vi "countrate_viewer_mpix.vi"() -> ()   [LabVIEW 2022 SP3]
uses:
  af06e324-2b0b-4744-b8ce-6f47c907ae65.vi
  <vilib>/Comparison/Less/Less Functor/Less Functor.lvclass
panel:
  in  "Thscan Folder Path":path=path "C:/Users/User/OneDrive/measurements/mpix/2023-04-14_pommiary_RK_testowe_przed_RG/0050mA/7a_ikrum=  2; igm= 32; vt0=  s; vt1=   ; DIS_DYN_SW= ; MPR_en= ; bgshc_W= ; bgshc_N= ; bgshc_NW= ;"
  in  "Current":u16(ring)=1 items=["0050mA", "0100mA", "0150mA"]
  in  "Tab Control":enum32{"Single pixel", "Pixels ROI"}(tab)
  out "Counns_vs_Current":cluster{i32[], i32[]}(graph)
  out "SP_Thscans":i32[][](graph)
  out "ROI_Thscans":i32[][](graph)
  out "ROI Counns_vs_Current":cluster{"x":i32[], "y":i32[]}[](graph)
  out "Image":i32[][](graph)
  in  "ThScan_Load":bool
  in  "Exit":bool
  # "counts vs. current for single pixel for single vt"
  # "thscans of all currents for single pixel"
  # "counts vs. current for ROI pixels for single vt"
  # "thscans of ROI pixels for single current"
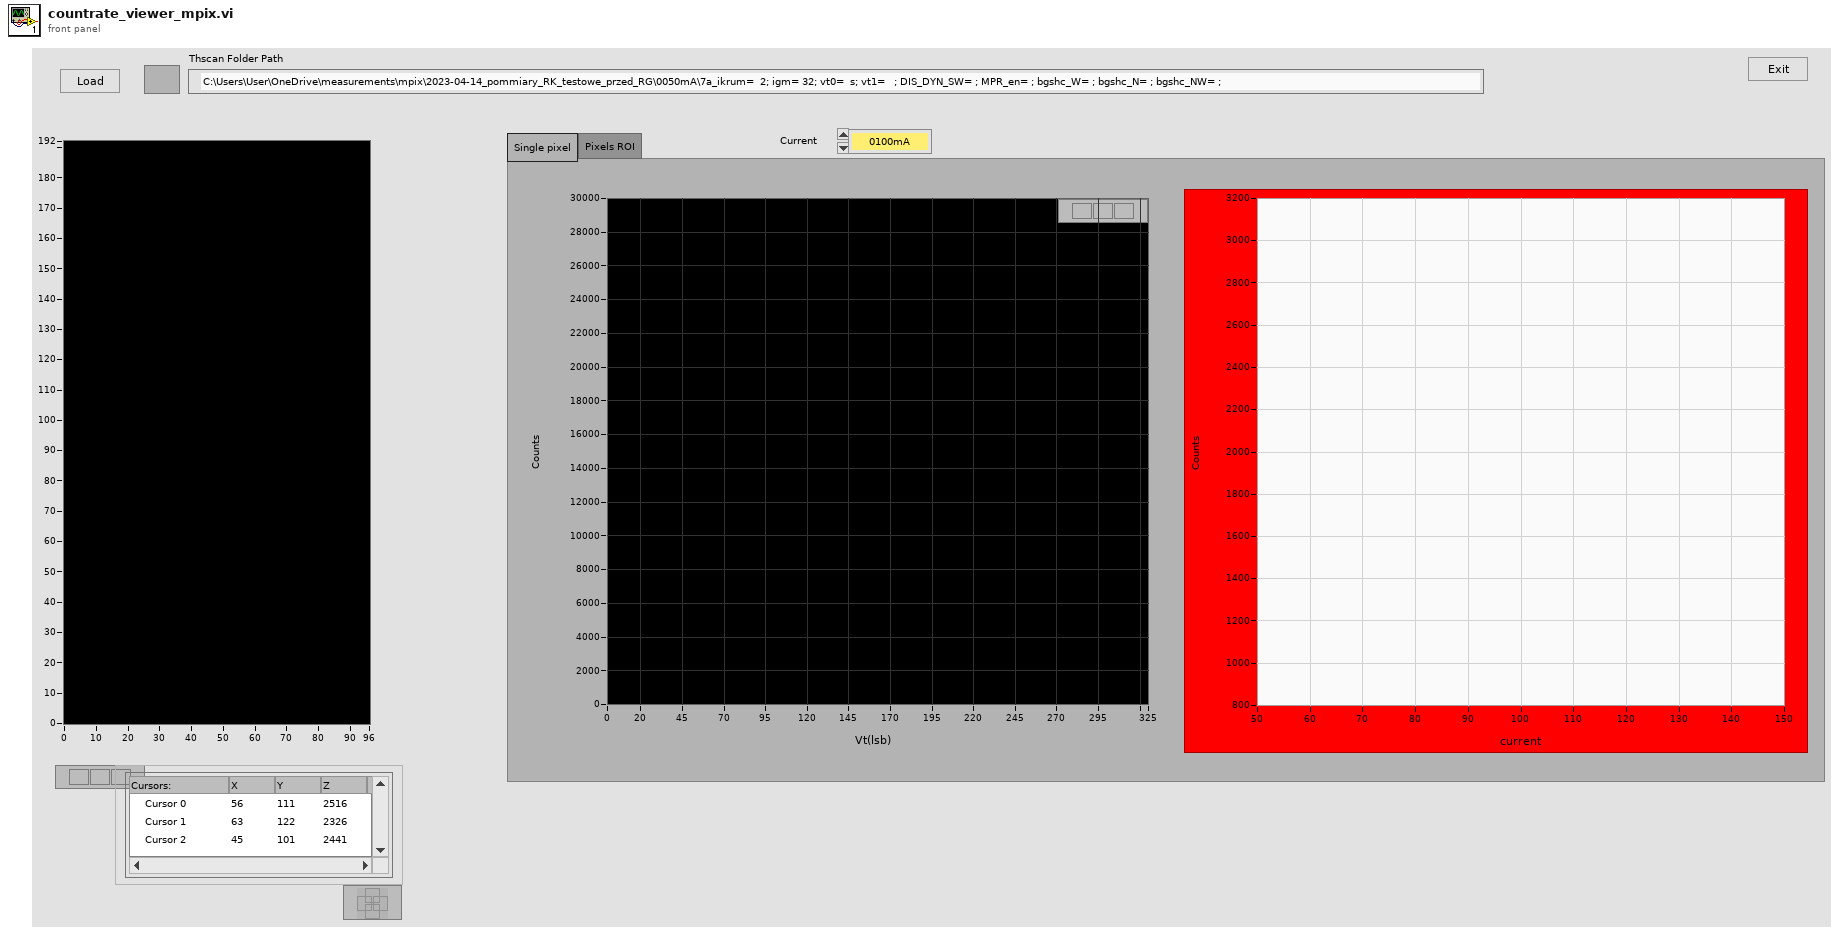
[diagram p1: front panel]
types:
  T1 = enum16{"big-endian, network order", "native, host order", "little-endian"}
  T2 = typedef "LVPointDoubleTypeDef.ctl" = cluster{"Cursor X":dbl, "Cursor Y":dbl}
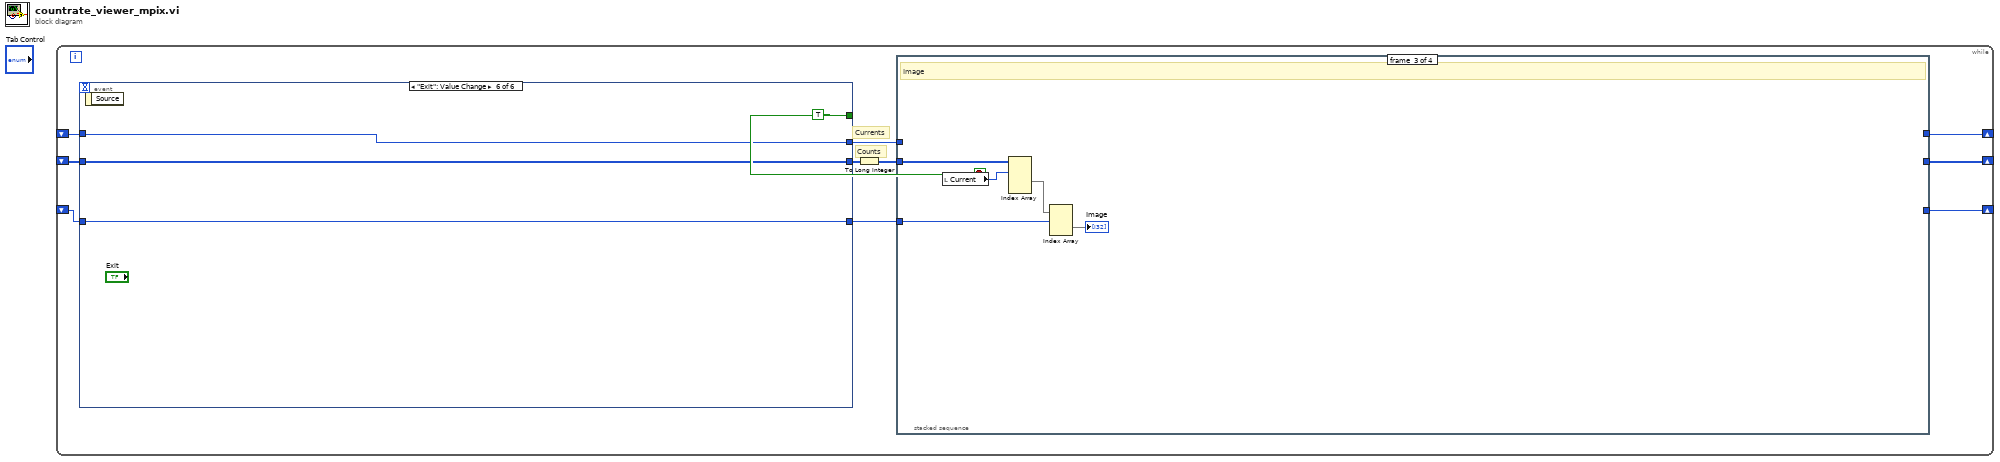
[diagram p0: block diagram]
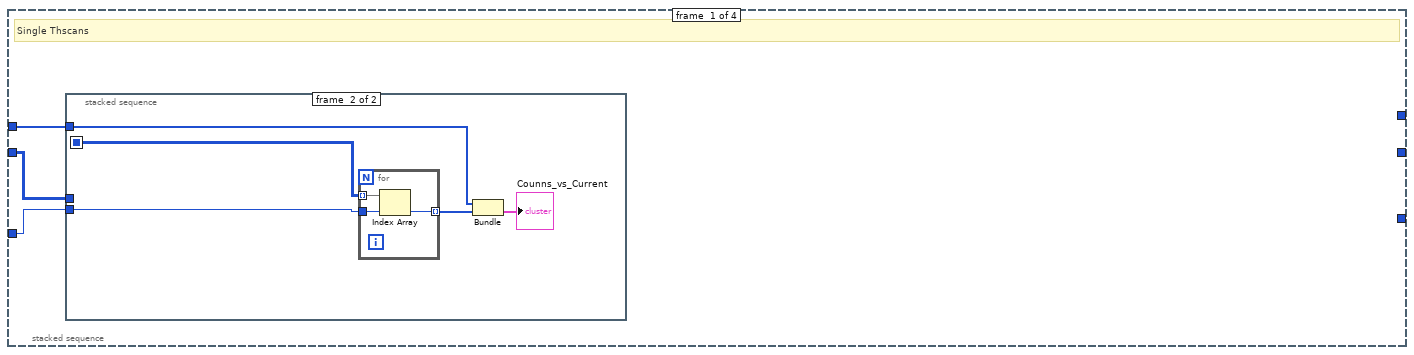
[diagram p2: hidden frame]
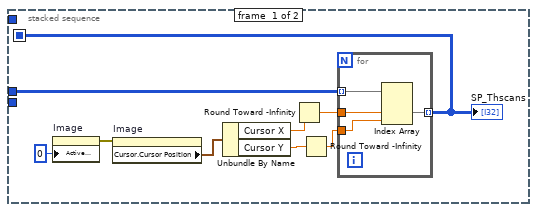
[diagram p3: hidden frame]
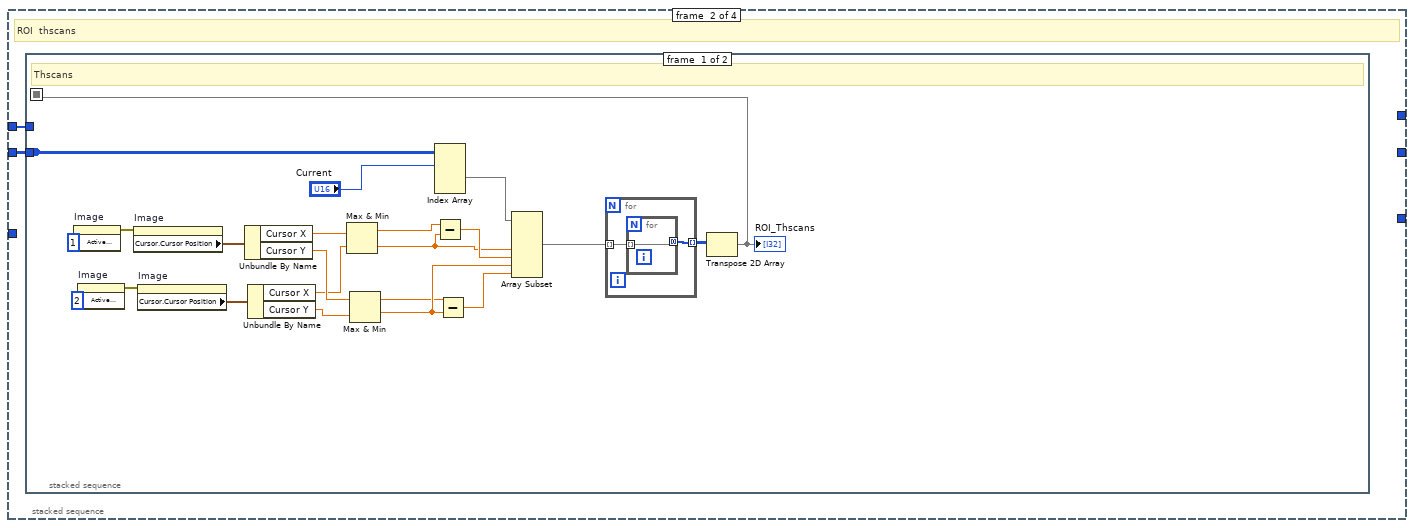
[diagram p4: hidden frame]
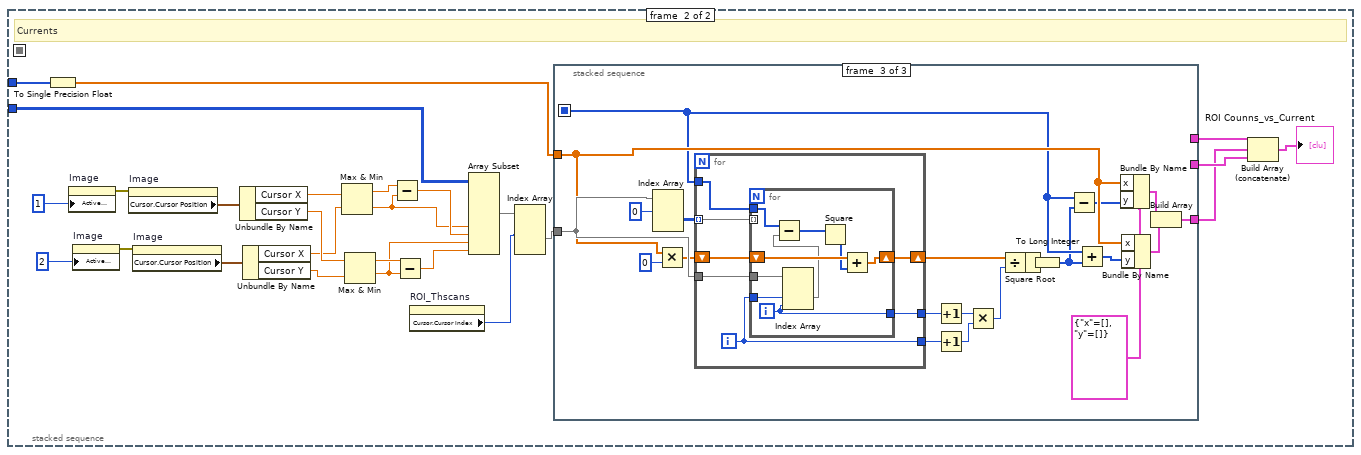
[diagram p5: hidden frame]
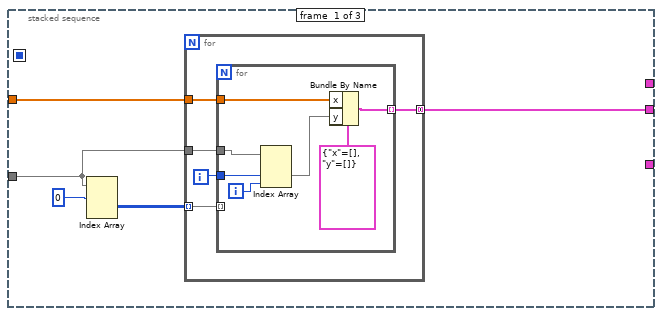
[diagram p6: hidden frame]
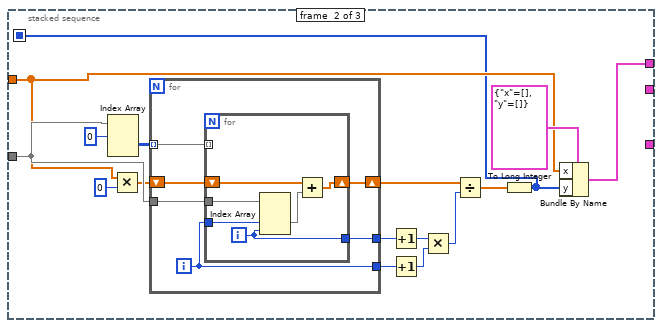
[diagram p7: hidden frame]
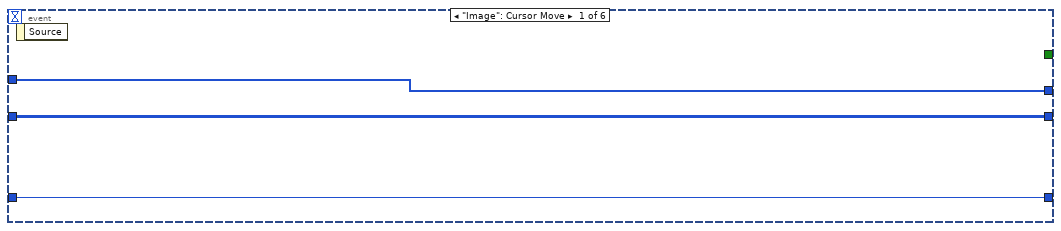
[diagram p9: hidden frame]
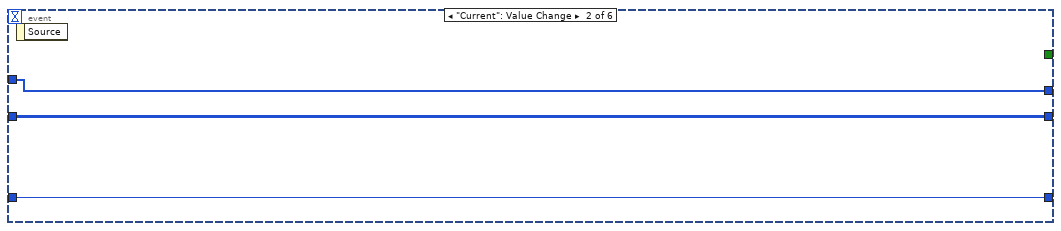
[diagram p10: hidden frame]
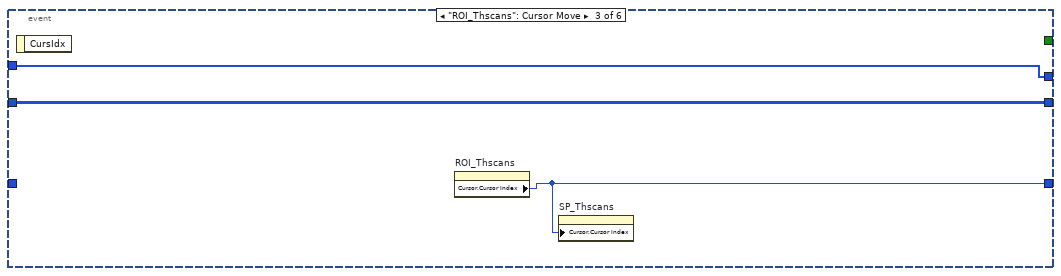
[diagram p11: hidden frame]
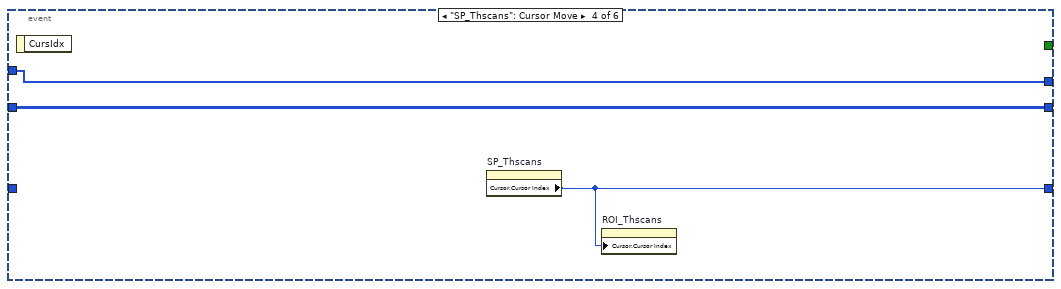
[diagram p12: hidden frame]
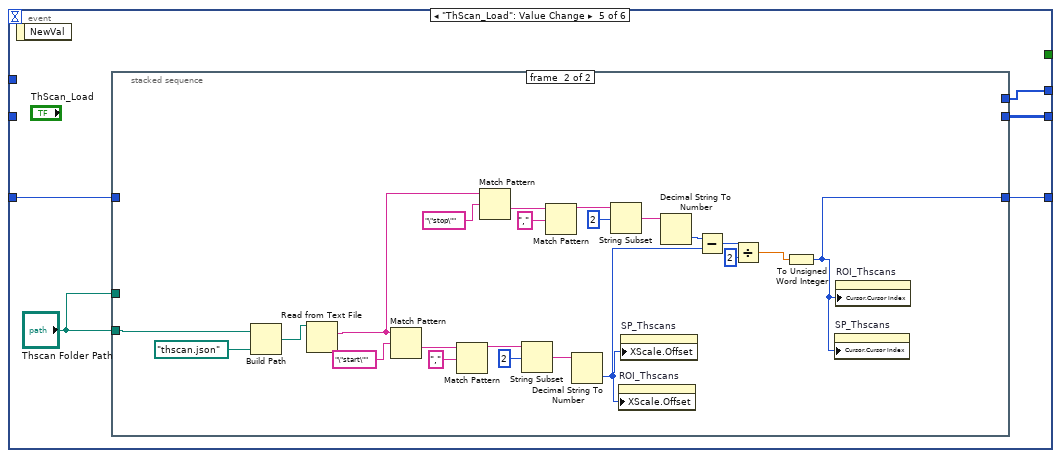
[diagram p13: hidden frame]
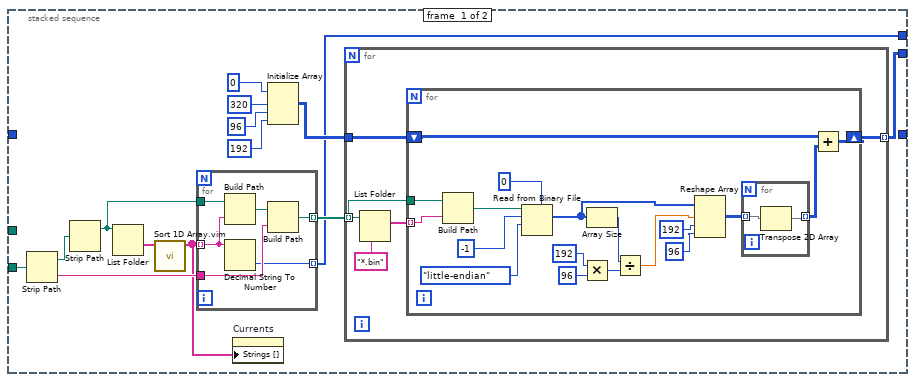
[diagram p14: hidden frame]
diagram:
  n1 = while {
    shift-right: [w8] -> _
    shift-left: _ -> [w10]
    shift-right: [w5] -> _
    shift-left: _ -> [w7]
    shift-right: [w2] -> _
    shift-left: _ -> [w1]
    stop <- w11 stop-if-true
    # "Counts"
    # "Currents"
    n2 = event shown="[5] \"Exit\": Value Change" {
      selector: _ -> [_ _ _ _ _ _]
      dyn-events: _ -> [_ _ _ _ _ _]
      timeout: _ -> [_ _ _ _ _ _]
      tunnel: [_ _ _ _ _ TRUE] -> w11
      tunnel: w10 -> [w182 w184 w188 w190 _ w266]
      tunnel: [w182 w184 w188 w190 w195 w266] -> w9
      tunnel: w7 -> [w181 w185 w187 w191 _ w265]
      tunnel: [w181 w185 w187 w191 w196 w265] -> w6
      tunnel: [w180 w183 w186 w189 w193 w264] -> w3
      tunnel: w1 -> [w180 w183 _ _ w192 w264]
      event "Image": Cursor Move {
        n3 = event-data() -> ()  [unwired: 1 in, 1 out]
      }
      event "Current": Value Change {
        n4 = event-data() -> ()  [unwired: 1 in, 1 out]
      }
      event "ROI_Thscans": Cursor Move {
        n5 = event-data() -> ()  [unwired: 1 in, 1 out]
        n6 = property on="ROI_Thscans" class="WFGraph (strict)"() -> ("Cursor.Cursor Index"=w186:i32)  [unwired: 2 in, 2 out]
        n7 = property on="SP_Thscans" class="WFGraph (strict)"("Cursor.Cursor Index"=w186) -> ()  [unwired: 2 in, 2 out]
      }
      event "SP_Thscans": Cursor Move {
        n8 = event-data() -> ()  [unwired: 1 in, 1 out]
        n9 = property on="SP_Thscans" class="WFGraph (strict)"() -> ("Cursor.Cursor Index"=w189:i32)  [unwired: 2 in, 2 out]
        n10 = property on="ROI_Thscans" class="WFGraph (strict)"("Cursor.Cursor Index"=w189) -> ()  [unwired: 2 in, 2 out]
      }
      event "ThScan_Load": Value Change {
        n11 = event-data() -> ()  [unwired: 1 in, 1 out]
        n12 = stacked-sequence {
          tunnel: [w200 _] -> w196
          tunnel: [w199 _] -> w195
          tunnel: "Thscan Folder Path" -> [w197 w255]
          tunnel: "Thscan Folder Path" -> [_ _]
          tunnel: [_ w243] -> w193
          tunnel: w192 -> [_ _]
          frame #0 {
            n13 = Strip Path(path=w197) -> (stripped path=w210:path, name=w208:string)
            n14 = Strip Path(path=w210) -> (stripped path=w207:path)  [unwired: 1 out]
            n15 = List Folder(path=w207) -> (folder names=w209:string[])  [unwired: 3 in, 3 out]
            n16 = call "Sort 1D Array.vim"("unsorted array"=w209) -> ("sorted array"=w198:string[])  [unwired: 10 in]
            n17 = for {
              tunnel: w198 -> [w237] mode=indexing
              tunnel: w208 -> [w239]
              tunnel: w207 -> [w241]
              tunnel: [w238] -> w206 mode=indexing
              tunnel: [w236] -> w200 mode=indexing
              n18 = Build Path(base path=w241, name or relative path=w237) -> (appended path=w240:path)
              n19 = Decimal String To Number(string=w237) -> (number=w236:i32)  [unwired: 2 in, 1 out]
              n20 = Build Path(base path=w240, name or relative path=w239) -> (appended path=w238:path)
            }
            n21 = property on="Currents" class="Ring (strict)"("Strings []"=w198) -> ()  [unwired: 2 in, 2 out]
            n22 = Initialize Array(u32 0 ("element"), 320, 96, 192) -> (w201:u32[][][])
            n23 = for {
              tunnel: w206 -> [w213] mode=indexing
              tunnel: [w212] -> w199 mode=indexing
              tunnel: w201 -> [w211]
              n24 = List Folder(path=w213, pattern="*.bin") -> (filenames=w214:string[])  [unwired: 2 in, 3 out]
              n25 = for {
                tunnel: w214 -> [w232] mode=indexing
                tunnel: w213 -> [w233]
                shift-right: [w216] -> w212
                shift-left: w211 -> [w218]
                n26 = Build Path(base path=w233, name or relative path=w232) -> (appended path=w219:path)
                n27 = Read from Binary File(5:u16 0, 9:T1."little-endian" ("byte order (0:big-endian, network order)"), 10:-1 ("count (1)"), 11:w219) -> (2:w228:u16[])  [unwired: 2 in, 3 out]
                n28 = Multiply(x=192 ("dimension size"), y=96 ("dimension size")) -> (x*y=w230:i32)
                n29 = Array Size(array=w228) -> (size(s)=w231:i32)
                n30 = Divide(x=w231, y=w230) -> (x/y=w229:dbl)
                n31 = Reshape Array(w228, w229, 192 ("dimension size"), 96 ("dimension size")) -> (w227:u16[][][])
                n32 = for {
                  tunnel: w227 -> [w235] mode=indexing
                  tunnel: [w234] -> w217 mode=indexing
                  n33 = Transpose 2D Array(2D array=w235) -> (transposed array=w234:u16[][])
                }
                n34 = Add(x=w218, y=w217) -> (x+y=w216:u32[][][])
              }
            }
          }
          frame #1 {
            n35 = Build Path(base path=w255, name or relative path=path "thscan.json") -> (appended path=w260:path)
            n36 = Read from Text File(file (use dialog)=w260) -> (text=w248:string)  [unwired: 3 in, 3 out]
            n37 = Match Pattern(string=w248, regular expression="\"start\"") -> (after substring=w261:string)  [unwired: 1 in, 3 out]
            n38 = Match Pattern(string=w261, regular expression=",") -> (before substring=w262:string)  [unwired: 1 in, 3 out]
            n39 = Match Pattern(string=w248, regular expression="\"stop\"") -> (after substring=w252:string)  [unwired: 1 in, 3 out]
            n40 = String Subset(string=w262, offset (0)=2) -> (substring=w263:string)  [unwired: 1 in]
            n41 = Match Pattern(string=w252, regular expression=",") -> (before substring=w253:string)  [unwired: 1 in, 3 out]
            n42 = Decimal String To Number(string=w263) -> (number=w244:i32)  [unwired: 2 in, 1 out]
            n43 = String Subset(string=w253, offset (0)=2) -> (substring=w254:string)  [unwired: 1 in]
            n44 = property on="ROI_Thscans" class="WFGraph (strict)"("XScale.Offset"=w244) -> ()  [unwired: 2 in, 2 out]
            n45 = property on="SP_Thscans" class="WFGraph (strict)"("XScale.Offset"=w244) -> ()  [unwired: 2 in, 2 out]
            n46 = Decimal String To Number(string=w254) -> (number=w247:i32)  [unwired: 2 in, 1 out]
            n47 = Subtract(x=w247, y=w244) -> (x-y=w246:i32)
            n48 = Divide(x=w246, y=2) -> (x/y=w242:dbl)
            n49 = To Unsigned Word Integer(number=w242) -> (unsigned 16bit integer=w243:u16)
            n50 = property on="SP_Thscans" class="WFGraph (strict)"("Cursor.Cursor Index"=w243) -> ()  [unwired: 2 in, 2 out]
            n51 = property on="ROI_Thscans" class="WFGraph (strict)"("Cursor.Cursor Index"=w243) -> ()  [unwired: 2 in, 2 out]
          }
        }
      }
      event "Exit": Value Change {
        n52 = event-data() -> ()  [unwired: 1 in, 1 out]
      }
    }
    n53 = To Long Integer(number=w9) -> (32bit integer=w4:i32[][][][])
    n54 = stacked-sequence {
      tunnel: w4 -> [w14 w37 w173 w179]
      tunnel: [_ _ _ w179] -> w8
      tunnel: w6 -> [w13 w36 _ w178]
      tunnel: [_ _ _ w178] -> w5
      tunnel: [_ w37 _ _] -> _
      tunnel: w3 -> [w12 _ w172 w177]
      tunnel: [_ _ _ w177] -> w2
      frame #0 {
        # "Single Thscans"
        n55 = stacked-sequence {
          seq-local: [w15 _] -> [_ w29]
          tunnel: w14 -> [w16 _]
          tunnel: w13 -> [_ w30]
          tunnel: w12 -> [_ w28]
          frame #0 {
            n56 = property on="Image" class="IntGraph (strict)"("Active Cursor"=u32 0) -> (error out=w18:errorcluster)  [unwired: 2 in, 1 out]
            n57 = property on="Image" class="IntGraph (strict)"(error in=w18) -> ("Cursor.Cursor Position"=w19:T2)  [unwired: 1 in, 2 out]
            n58 = Unbundle By Name(w19) -> ("Cursor X"=w21:dbl, "Cursor Y"=w22:dbl)
            n59 = Round Toward -Infinity(1:w21) -> (0:w20:dbl)
            n60 = Round Toward -Infinity(1:w22) -> (0:w23:dbl)
            n61 = for {
              tunnel: w23 -> [w27]
              tunnel: w20 -> [w26]
              tunnel: w16 -> [w25] mode=indexing
              tunnel: [w24] -> w15 mode=indexing
              n62 = Index Array(array=w25, index (dim 1)=w26, index (dim 2)=w27) -> (element=w24:i32[])  [unwired: 1 in]
            }
            "SP_Thscans" <- w15
          }
          frame #1 {
            n63 = for {
              tunnel: w29 -> [w35] mode=indexing
              tunnel: w28 -> [w34]
              tunnel: [w33] -> w31 mode=indexing
              n64 = Index Array(array=w35, index=w34) -> (element=w33:i32)
            }
            n65 = Bundle(w30, w31) -> (→"Counns_vs_Current":cluster{i32[], i32[]})  [unwired: 1 in]
          }
        }
      }
      frame #1 {
        # "ROI  thscans"
        n66 = stacked-sequence {
          seq-local: [w38 _] -> [_ _]
          tunnel: w37 -> [w39 w76]
          tunnel: w36 -> [_ w69]
          frame #0 {
            # "Thscans"
            n67 = property on="Image" class="IntGraph (strict)"("Active Cursor"=u32 1) -> (error out=w46:errorcluster)  [unwired: 2 in, 1 out]
            n68 = property on="Image" class="IntGraph (strict)"("Active Cursor"=u32 2) -> (error out=w47:errorcluster)  [unwired: 2 in, 1 out]
            n69 = property on="Image" class="IntGraph (strict)"(error in=w46) -> ("Cursor.Cursor Position"=w48:T2)  [unwired: 1 in, 2 out]
            n70 = property on="Image" class="IntGraph (strict)"(error in=w47) -> ("Cursor.Cursor Position"=w49:T2)  [unwired: 1 in, 2 out]
            n71 = Unbundle By Name(w48) -> ("Cursor X"=w50:dbl, "Cursor Y"=w52:dbl)
            n72 = Unbundle By Name(w49) -> ("Cursor X"=w51:dbl, "Cursor Y"=w53:dbl)
            n73 = Max & Min(x=w50, y=w51) -> (max(x,y)=w54:dbl, min(x,y)=w55:dbl)
            n74 = Max & Min(x=w52, y=w53) -> (max(x,y)=w57:dbl, min(x,y)=w59:dbl)
            n75 = Index Array(array=w39, index (dim 0)="Current") -> (element=w41:i32[][][])  [unwired: 3 in]
            n76 = Subtract(x=w54, y=w55) -> (x-y=w56:dbl)
            n77 = Subtract(x=w57, y=w59) -> (x-y=w58:dbl)
            n78 = Array Subset(array=w41, index (dim 1)=w55, length (dim 1)=w56, index (dim 2)=w59, length (dim 2)=w58) -> (w45:i32[][][])  [unwired: 2 in]
            n79 = for {
              tunnel: [w61] -> w44 mode=indexing
              tunnel: w45 -> [w60] mode=indexing
              n80 = for {
                tunnel: w60 -> [w62] mode=indexing
                tunnel: [w62] -> w61 mode=concatenating
              }
            }
            n81 = Transpose 2D Array(2D array=w44) -> (transposed array=w38:i32[][])
            "ROI_Thscans" <- w38
          }
          frame #1 {
            # "Currents"
            n82 = To Single Precision Float(number=w69) -> (single precision float=w63:sgl[])
            n83 = property on="Image" class="IntGraph (strict)"("Active Cursor"=u32 1) -> (error out=w79:errorcluster)  [unwired: 2 in, 1 out]
            n84 = property on="Image" class="IntGraph (strict)"("Active Cursor"=u32 2) -> (error out=w80:errorcluster)  [unwired: 2 in, 1 out]
            n85 = property on="Image" class="IntGraph (strict)"(error in=w79) -> ("Cursor.Cursor Position"=w81:T2)  [unwired: 1 in, 2 out]
            n86 = property on="Image" class="IntGraph (strict)"(error in=w80) -> ("Cursor.Cursor Position"=w82:T2)  [unwired: 1 in, 2 out]
            n87 = Unbundle By Name(w81) -> ("Cursor X"=w83:dbl, "Cursor Y"=w85:dbl)
            n88 = Unbundle By Name(w82) -> ("Cursor X"=w84:dbl, "Cursor Y"=w86:dbl)
            n89 = Max & Min(x=w83, y=w84) -> (max(x,y)=w87:dbl, min(x,y)=w72:dbl)
            n90 = Max & Min(x=w85, y=w86) -> (max(x,y)=w88:dbl, min(x,y)=w74:dbl)
            n91 = Subtract(x=w87, y=w72) -> (x-y=w73:dbl)
            n92 = Subtract(x=w88, y=w74) -> (x-y=w75:dbl)
            n93 = property on="ROI_Thscans" class="WFGraph (strict)"() -> ("Cursor.Cursor Index"=w68:i32)  [unwired: 2 in, 2 out]
            n94 = Array Subset(array=w76, index (dim 2)=w72, length (dim 2)=w73, index (dim 3)=w74, length (dim 3)=w75) -> (w71:i32[][][][])  [unwired: 4 in]
            n95 = Index Array(array=w71, index (dim 1)=w68) -> (element=w70:i32[][][])  [unwired: 3 in]
            n96 = stacked-sequence {
              seq-local: [_ w106 _] -> [_ _ w141]
              tunnel: w70 -> [w91 w113 w150]
              tunnel: w63 -> [w90 w111 w142]
              tunnel: [w89 _ _] -> w66
              tunnel: [_ w120 _] -> w65
              tunnel: [_ _ w137] -> w64
              frame #0 {
                n97 = Index Array(array=w91, index (dim 0)=0 ("index (page)")) -> (element=w92:i32[][])  [unwired: 2 in]
                n98 = for {
                  tunnel: w92 -> [w98] mode=indexing
                  tunnel: w91 -> [w97]
                  tunnel: w90 -> [w95]
                  tunnel: [w94] -> w89 mode=concatenating
                  i -> [w96]
                  n99 = for {
                    tunnel: w98 -> [_] mode=indexing
                    tunnel: w97 -> [w105]
                    tunnel: w96 -> [w103]
                    tunnel: w95 -> [w101]
                    tunnel: [w99] -> w94 mode=indexing
                    i -> [w104]
                    n100 = Index Array(array=w105, index (dim 1)=w103, index (dim 2)=w104) -> (element=w100:i32[])  [unwired: 1 in]
                    n101 = Bundle By Name(cluster=cluster{"x":i32[], "y":i32[]} {"x"=[], "y"=[]}, "x"=w101, "y"=w100) -> (w99:cluster{"x":i32[], "y":i32[]})
                  }
                }
              }
              frame #1 {
                n102 = Index Array(array=w113, index (dim 0)=0 ("index (page)")) -> (element=w112:i32[][])  [unwired: 2 in]
                n103 = Multiply(x=w111, y=0 ("index (page)")) -> (x*y=w110:sgl[])
                n104 = for {
                  tunnel: w113 -> [w127]
                  shift-right: [w125] -> w115
                  shift-left: w110 -> [w126]
                  tunnel: [w124] -> w119
                  tunnel: [w123] -> w118
                  tunnel: w112 -> [w122] mode=indexing
                  i -> [w123]
                  n105 = for {
                    tunnel: w127 -> [w131]
                    shift-right: [w133] -> w125
                    shift-left: w126 -> [w132]
                    tunnel: [w128] -> w124
                    tunnel: w123 -> [w129]
                    tunnel: w122 -> [_] mode=indexing
                    i -> [w128]
                    n106 = Index Array(array=w131, index (dim 1)=w129, index (dim 2)=w128) -> (element=w130:i32[])  [unwired: 1 in]
                    n107 = Add(x=w132, y=w130) -> (x+y=w133:sgl[])
                  }
                }
                n108 = Increment(x=w119) -> (x+1=w108:i32)
                n109 = Increment(x=w118) -> (x+1=w107:i32)
                n110 = Multiply(x=w108, y=w107) -> (x*y=w117:i32)
                n111 = Divide(x=w115, y=w117) -> (x/y=w116:sgl[])
                n112 = To Long Integer(number=w116) -> (32bit integer=w106:i32[])
                n113 = Bundle By Name(cluster=cluster{"x":i32[], "y":i32[]} {"x"=[], "y"=[]}, "x"=w111, "y"=w106) -> (w120:cluster{"x":i32[], "y":i32[]})
              }
              frame #2 {
                w143 = cluster{"x":i32[], "y":i32[]} {"x"=[], "y"=[]}
                n114 = Index Array(array=w150, index (dim 0)=0 ("index (page)")) -> (element=w149:i32[][])  [unwired: 2 in]
                n115 = Multiply(x=w142, y=0 ("index (page)")) -> (x*y=w148:sgl[])
                n116 = for {
                  tunnel: w150 -> [w162]
                  shift-right: [w160] -> w152
                  shift-left: w148 -> [w161]
                  tunnel: [w159] -> w155
                  tunnel: [w158] -> w154
                  tunnel: w149 -> [w157] mode=indexing
                  tunnel: w141 -> [w156]
                  i -> [w158]
                  n117 = for {
                    tunnel: w162 -> [w169]
                    shift-right: [w171] -> w160
                    shift-left: w161 -> [w170]
                    tunnel: [w167] -> w159
                    tunnel: w158 -> [w168]
                    tunnel: w157 -> [_] mode=indexing
                    tunnel: w156 -> [w166]
                    i -> [w167]
                    n118 = Index Array(array=w169, index (dim 1)=w168, index (dim 2)=w167) -> (element=w165:i32[])  [unwired: 1 in]
                    n119 = Subtract(x=w166, y=w165) -> (x-y=w164:i32[])
                    n120 = Square(x=w164) -> (x^2=w163:i32[])
                    n121 = Add(x=w170, y=w163) -> (x+y=w171:sgl[])
                  }
                }
                n122 = Increment(x=w155) -> (x+1=w146:i32)
                n123 = Increment(x=w154) -> (x+1=w145:i32)
                n124 = Multiply(x=w146, y=w145) -> (x*y=w153:i32)
                n125 = Divide(x=w152, y=w153) -> (x/y=w135:sgl[])
                n126 = Square Root(x=w135) -> (sqrt(x)=w134:sgl[])
                n127 = To Long Integer(number=w134) -> (32bit integer=w140:i32[])
                n128 = Subtract(x=w141, y=w140) -> (x-y=w139:i32[])
                n129 = Add(x=w141, y=w140) -> (x+y=w144:i32[])
                n130 = Bundle By Name(cluster=w143, "x"=w142, "y"=w139) -> (w138:cluster{"x":i32[], "y":i32[]})
                n131 = Bundle By Name(cluster=w143, "x"=w142, "y"=w144) -> (w136:cluster{"x":i32[], "y":i32[]})
                n132 = Build Array(w138, w136) -> (w137:cluster{"x":i32[], "y":i32[]}[])
              }
            }
            n133 = Build Array (concatenate)(w65, w64, w66) -> (→"ROI Counns_vs_Current":cluster{"x":i32[], "y":i32[]}[])
          }
        }
      }
      frame #2 {
        # "Image"
        n134 = local read "Current"() -> (w175:u16)
        n135 = Index Array(array=w173, index (dim 0)=w175) -> (element=w174:i32[][][])  [unwired: 3 in]
        n136 = Index Array(array=w174, index (dim 0)=w172) -> (element=→"Image":i32[][])  [unwired: 2 in]
      }
      frame #3 {
      }
    }
  }
